vi "CRYEqual DataView Idx and Actived Wnd.vi"() -> (0 "DataView QueueName":string, 2 "bResult":bool, 3 "DataView Index":i32)   [LabVIEW 2013]
uses:
  CRYNew View Global.vi
  SubVI/CRYMain Sub Window Global.vi
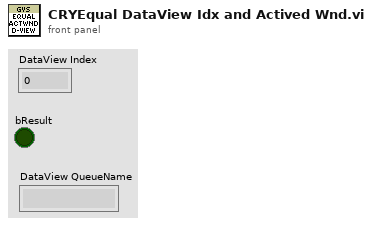
[diagram p1: front panel]
types:
  T1 = typedef "Graph Main Info Cluster.ctl" = cluster{"Selected_BarIdx":i32, "Selected_PanelIdx":i32, "Graph Main VIRef":refnum<vi>, "ToolBarClick":bool, "Spliter Ref Array":refnum<vi>[], "Panel Ref Array":refnum<vi>[], "Spliter_matrix":i32[][], "Panel_matrix":i32[][], "child_spliterIdx_matrix":i32[][], "split_pos_matrix":i32[][], "Title State":bool, "sQueueName":string, "Frame nID":i32, "Graph VIRef Array":cluster{"Graph VIRef":refnum<vi>, "Panel Idx":i32, "Frame VIRef":refnum<vi>, "Icon Ring":i32, "Graph Type":string}[], "View Type":string}
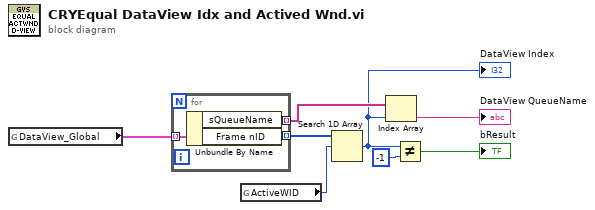
[diagram p0: block diagram]
diagram:
  n1 = global read "CRYNew View Global.vi" "DataView_Global"() -> (w4:T1[])
  n2 = for {
    tunnel: [w11] -> w7 mode=indexing
    tunnel: w4 -> [w10] mode=indexing
    tunnel: [w9] -> w3 mode=indexing
    n3 = Unbundle By Name(w10) -> ("sQueueName"=w9:string, "Frame nID"=w11:i32)
  }
  n4 = global read "CRYMain Sub Window Global.vi" "ActiveWID"() -> (w6:i32)
  n5 = Search 1D Array(1D array=w7, element=w6) -> (index of element=w2:i32)  [unwired: 1 in]
  "DataView Index" <- w2
  n6 = Index Array(array=w3, index=w2) -> (element=→"DataView QueueName":string)
  n7 = Not Equal?(x=w2, y=-1) -> (x != y?=→"bResult":bool)
